vi "generate random code.vi"() -> (3 "random code":string)   [LabVIEW 2013]
panel:
  out "十进制整型字符串":string
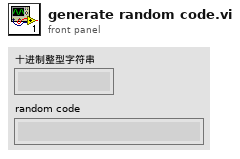
[diagram p1: front panel]
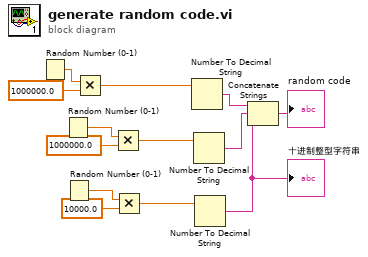
[diagram p0: block diagram]
diagram:
  n1 = Random Number (0-1)() -> (number: 0 to 1=w13:dbl)
  n2 = Random Number (0-1)() -> (number: 0 to 1=w11:dbl)
  n3 = Random Number (0-1)() -> (number: 0 to 1=w4:dbl)
  n4 = Multiply(x=w13, y=1000000.0) -> (x*y=w9:dbl)
  n5 = Multiply(x=w11, y=1000000.0) -> (x*y=w8:dbl)
  n6 = Multiply(x=w4, y=10000.0) -> (x*y=w2:dbl)
  n7 = Number To Decimal String(number=w9) -> (decimal integer string=w7:string)  [unwired: 1 in]
  n8 = Number To Decimal String(number=w8) -> (decimal integer string=w6:string)  [unwired: 1 in]
  n9 = Number To Decimal String(number=w2) -> (decimal integer string=w1:string)  [unwired: 1 in]
  "十进制整型字符串" <- w1
  n10 = Concatenate Strings(w7, w6, w1) -> (→"random code":string)
